vi "observerRegistry.vi"(7 "Action":T1(ring), 8 "error in":errorcluster, 9 "ObservableValue":variant[](array[variant]), 10 "ObservableName":string[](array[string])) -> (0 "error out":errorcluster, 3 "Observable out":T2(c390), 4 "size":i32)   [LabVIEW 2025, in "ObserverClass.lvlib"]
doc: "Handle Observer for each ObservableData available in application"
uses:
  ObserverClass.lvlib
  ObserverClass/Controls/observerControl.ctl
  ObserverClass/ObserverClass.lvclass
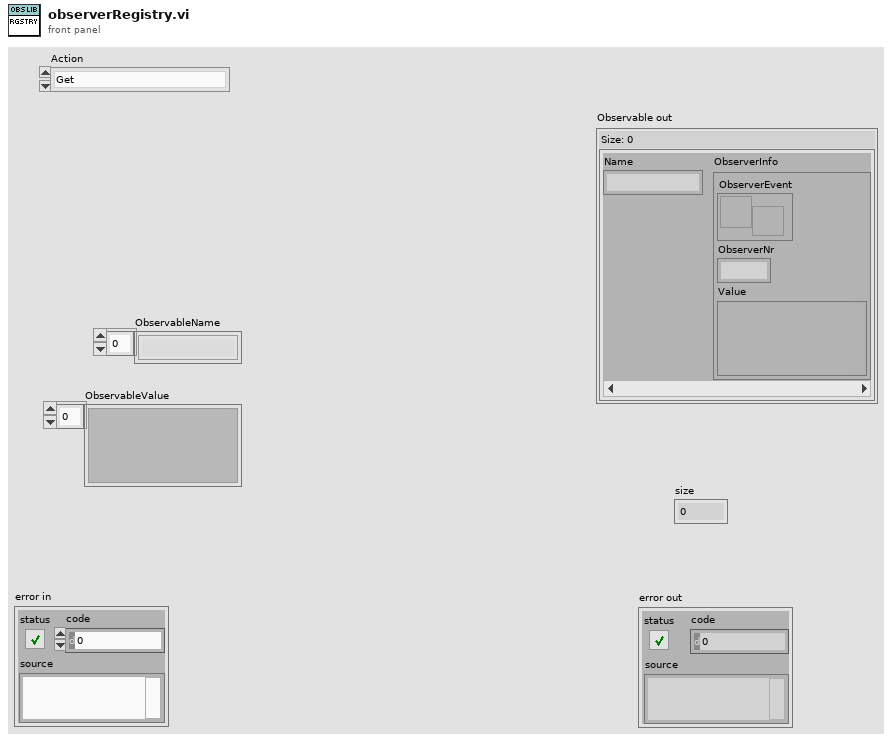
[diagram p1: front panel]
types:
  T1 = enum16{"Get", "Set", "Init", "Remove", "Destroy"}
  T2 = map{string, cluster{"ObserverEvent":refnum<user-event>, "ObserverNr":u64, "Value":variant}}
  T3 = cluster{"ObserverEvent":refnum<user-event>, "ObserverNr":u64, "Value":variant}
  T4 = typedef "ObserverClass.lvlib/ObserverClass.lvclass/observerControl.ctl" = cluster{"ObservableName":string, "ObservableValue":variant, "SenderName":string}
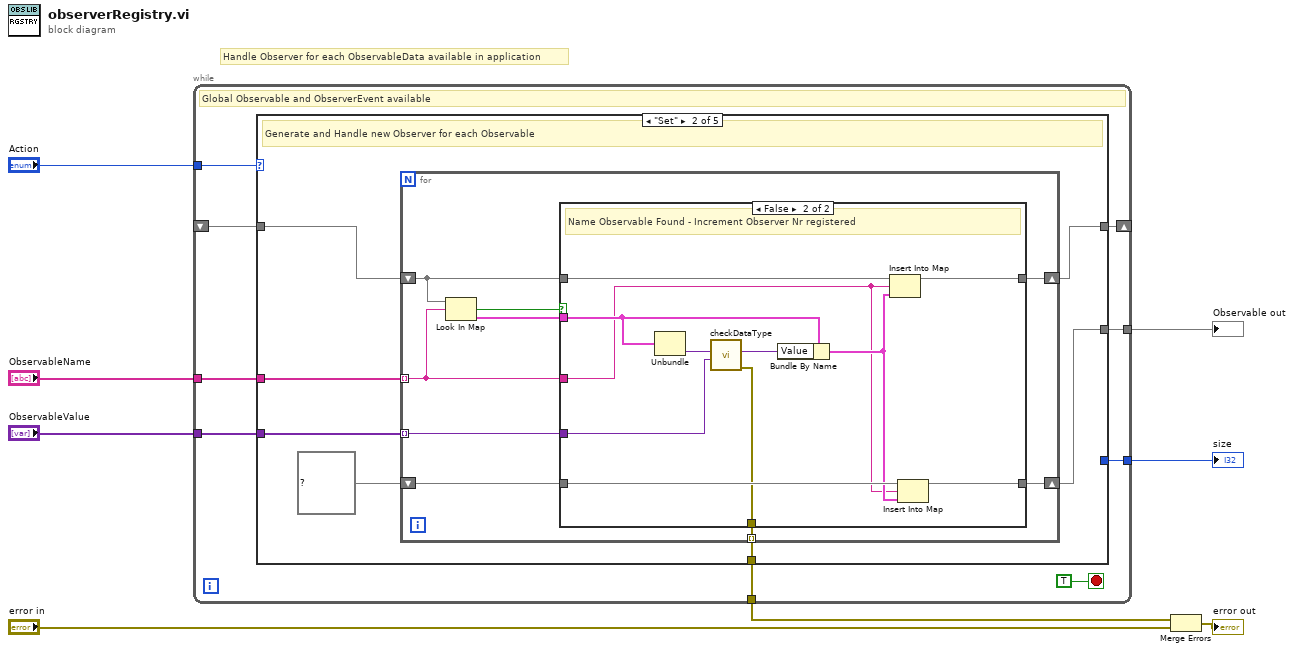
[diagram p0: block diagram]
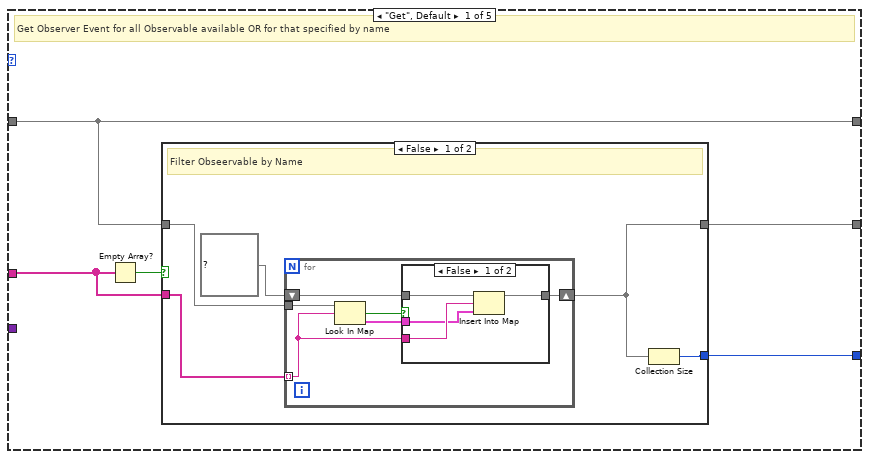
[diagram p2: hidden frame]
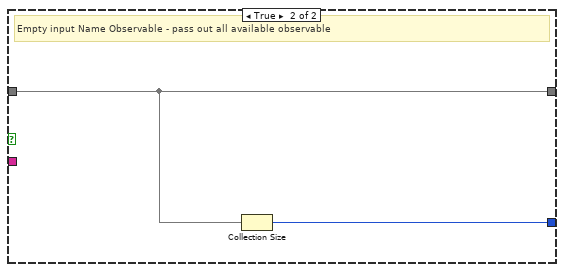
[diagram p4: hidden frame]
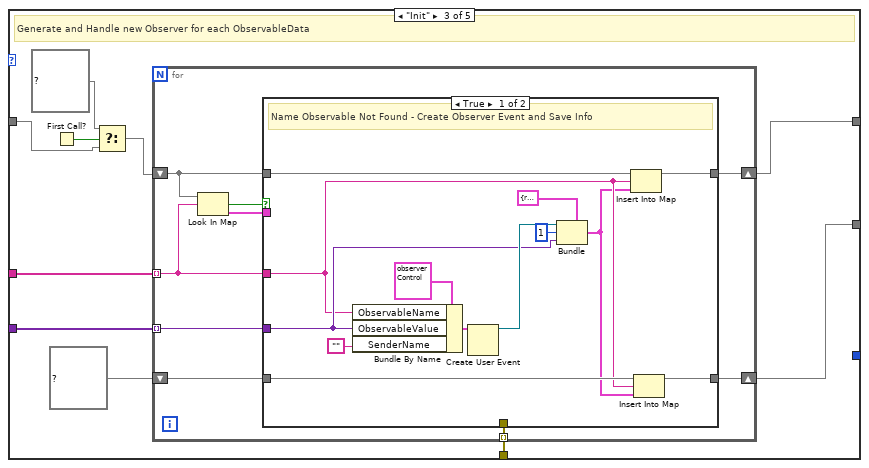
[diagram p6: hidden frame]
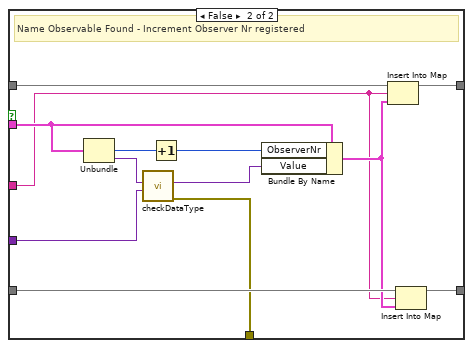
[diagram p7: hidden frame]
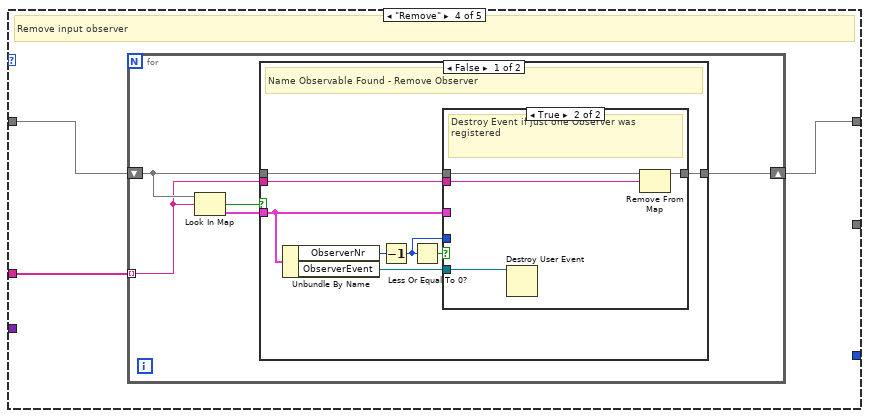
[diagram p8: hidden frame]
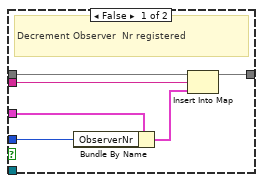
[diagram p9: hidden frame]
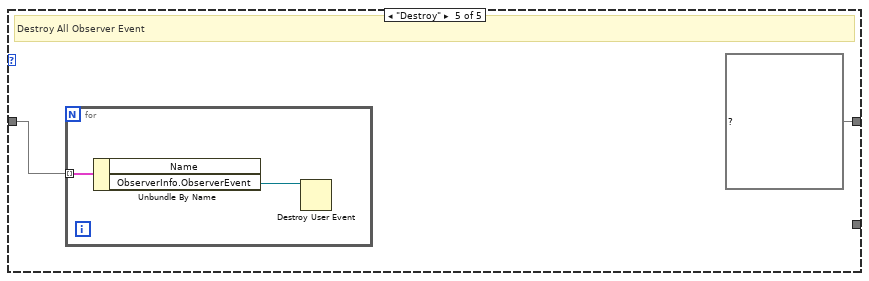
[diagram p11: hidden frame]
diagram:
  # "Handle Observer for each ObservableData available in application"
  n1 = while {
    tunnel: "ObservableName" -> [w17]
    tunnel: "ObservableValue" -> [w16]
    shift-right: [w13] -> _
    shift-left: _ -> [w14]
    tunnel: "Action" -> [w12]
    tunnel: [w11] -> w8
    tunnel: [w10] -> w3
    tunnel: [w9] -> w1
    stop <- TRUE stop-if-true
    # "Global Observable and ObserverEvent available"
    n2 = case shown="\"Set\"" w12 {
      tunnel: w17 -> [w20 w47 w79 w115 _]
      tunnel: w16 -> [_ w46 w78 _ _]
      tunnel: w14 -> [w19 w43 w72 w117 w143]
      tunnel: [w19 w45 w77 w116 T2 {} ("LiveData")] -> w13
      tunnel: [w22 _ _ _ _] -> w11
      tunnel: [w18 w44 w76 _ _] -> w10
      tunnel: [_ w41 w70 _ _] -> w9
      frame "Get", Default {
        # "Get Observer Event for all Observable available OR for that specified by name"
        n3 = Empty Array?(array=w20) -> (empty?=w21:bool)
        n4 = case shown="False" w21 {
          tunnel: [w25 w40] -> w22
          tunnel: w19 -> [w27 w39]
          tunnel: w20 -> [w26 _]
          tunnel: [w24 w39] -> w18
          frame False {
            # "Filter Obseervable by Name"
            n5 = for {
              tunnel: w26 -> [w32] mode=indexing
              tunnel: w27 -> [w33]
              shift-right: [w30] -> w24
              shift-left: T2 {} ("LiveData") -> [w29]
              n6 = Look In Map(map=w33, key=w32) -> (key not found?=w28:bool, value=w31:T3)  [unwired: 1 in]
              n7 = case shown="False" w28 {
                tunnel: w32 -> [w37 _]
                tunnel: w31 -> [w36 _]
                tunnel: [w35 w38] -> w30
                tunnel: w29 -> [w34 w38]
                frame False {
                  n8 = Insert Into Map(map in=w34, key=w37, value=w36) -> (map out=w35:T2)  [unwired: 2 out]
                }
                frame True {
                }
              }
            }
            n9 = Collection Size(1:w24) -> (0:w25:i32)
          }
          frame True {
            # "Empty input Name Observable - pass out all available observable"
            n10 = Collection Size(1:w39) -> (0:w40:i32)
          }
        }
      }
      frame "Set" {
        # "Generate and Handle new Observer for each Observable"
        n11 = for {
          tunnel: w47 -> [w53] mode=indexing
          tunnel: w46 -> [w56] mode=indexing
          shift-right: [w55] -> w45
          shift-left: w43 -> [w54]
          shift-right: [w49] -> w44
          shift-left: T2 {} ("LiveData") -> [w50]
          tunnel: [w48] -> w41 mode=indexing
          n12 = Look In Map(map=w54, key=w53) -> (key not found?=w52:bool, value=w51:T3)  [unwired: 1 in]
          n13 = case shown="False" w52 {
            tunnel: w56 -> [_ w60]
            tunnel: [w58 w67] -> w55
            tunnel: w54 -> [w58 w69]
            tunnel: w53 -> [_ w63]
            tunnel: w51 -> [_ w68]
            tunnel: w50 -> [w57 w66]
            tunnel: [w57 w65] -> w49
            tunnel: [_ w59] -> w48
            frame True {
              # "Name Observable Not Found - Do Nothing"
            }
            frame False {
              # "Name Observable Found - Increment Observer Nr registered"
              n14 = Unbundle(w68) -> ("Value"=w61:variant)  [unwired: 2 out]
              n15 = call "checkDataType.vi"("Data"=w60, "DataType"=w61) -> ("error out"=w59:errorcluster, "Data out"=w62:variant)  [unwired: 8 in]
              n16 = Bundle By Name(cluster=w68, "Value"=w62) -> (w64:T3)
              n17 = Insert Into Map(map in=w69, key=w63, value=w64) -> (map out=w67:T2)  [unwired: 2 out]
              n18 = Insert Into Map(map in=w66, key=w63, value=w64) -> (map out=w65:T2)  [unwired: 2 out]
            }
          }
        }
      }
      frame "Init" {
        # "Generate and Handle new Observer for each ObservableData"
        n19 = First Call?() -> (First Call?: T/F=w75:bool)
        n20 = Select(t=T2 {} ("LiveData"), s=w75, f=w72) -> (s? t:f=w73:T2)
        n21 = for {
          tunnel: w79 -> [w85] mode=indexing
          tunnel: w78 -> [w88] mode=indexing
          shift-right: [w87] -> w77
          shift-left: w73 -> [w86]
          shift-right: [w81] -> w76
          shift-left: T2 {} ("LiveData") -> [w82]
          tunnel: [w80] -> w70 mode=indexing
          n22 = Look In Map(map=w86, key=w85) -> (key not found?=w84:bool, value=w83:T3)  [unwired: 1 in]
          n23 = case shown="True" w84 {
            tunnel: w88 -> [w94 w103]
            tunnel: [w93 w110] -> w87
            tunnel: w86 -> [w98 w114]
            tunnel: w85 -> [w90 w106]
            tunnel: w83 -> [_ w113]
            tunnel: w82 -> [w92 w109]
            tunnel: [w91 w108] -> w81
            tunnel: [_ w102] -> w80
            frame True {
              # "Name Observable Not Found - Create Observer Event and Save Info"
              n24 = Bundle By Name(cluster=T4 {"ObservableName"="", "ObservableValue"=variant, "SenderName"=""} ("Observer"), "ObservableName"=w90, "ObservableValue"=w94, "SenderName"="") -> (w101:T4)
              n25 = Create User Event(user event datatype=w101) -> (user event=w97:refnum<user-event>)  [unwired: 1 in, 1 out]
              n26 = Bundle(cluster=T3 {"ObserverEvent"=refnum, "ObserverNr"=0, "Value"=variant} ("value"), "ObserverEvent"=w97, "ObserverNr"=u64 1, "Value"=w94) -> (w89:T3)
              n27 = Insert Into Map(map in=w98, key=w90, value=w89) -> (map out=w93:T2)  [unwired: 2 out]
              n28 = Insert Into Map(map in=w92, key=w90, value=w89) -> (map out=w91:T2)  [unwired: 2 out]
            }
            frame False {
              # "Name Observable Found - Increment Observer Nr registered"
              n29 = Unbundle(w113) -> ("ObserverNr"=w112:u64, "Value"=w104:variant)  [unwired: 1 out]
              n30 = call "checkDataType.vi"("Data"=w103, "DataType"=w104) -> ("error out"=w102:errorcluster, "Data out"=w105:variant)  [unwired: 8 in]
              n31 = Increment(x=w112) -> (x+1=w111:u64)
              n32 = Bundle By Name(cluster=w113, "ObserverNr"=w111, "Value"=w105) -> (w107:T3)
              n33 = Insert Into Map(map in=w114, key=w106, value=w107) -> (map out=w110:T2)  [unwired: 2 out]
              n34 = Insert Into Map(map in=w109, key=w106, value=w107) -> (map out=w108:T2)  [unwired: 2 out]
            }
          }
        }
      }
      frame "Remove" {
        # "Remove input observer"
        n35 = for {
          shift-right: [w122] -> w116
          shift-left: w117 -> [w121]
          tunnel: w115 -> [w120] mode=indexing
          n36 = Look In Map(map=w121, key=w120) -> (key not found?=w118:bool, value=w119:T3)  [unwired: 1 in]
          n37 = case shown="False" w118 {
            tunnel: [w130 w141] -> w122
            tunnel: w121 -> [w129 w141]
            tunnel: w120 -> [w127 _]
            tunnel: w119 -> [w125 _]
            frame False {
              # "Name Observable Found - Remove Observer"
              n38 = Unbundle By Name(w125) -> ("ObserverNr"=w124:u64, "ObserverEvent"=w128:refnum<user-event>)
              n39 = Decrement(x=w124) -> (x-1=w123:u64)
              n40 = Less Or Equal To 0?(x=w123) -> (x <= 0?=w126:bool)
              n41 = case shown="True" w126 {
                tunnel: [w136 w140] -> w130
                tunnel: w129 -> [w135 w139]
                tunnel: w128 -> [_ w138]
                tunnel: w127 -> [w134 w137]
                tunnel: w125 -> [w133 _]
                tunnel: w123 -> [w132 _]
                frame False {
                  # "Decrement Observer  Nr registered"
                  n42 = Bundle By Name(cluster=w133, "ObserverNr"=w132) -> (w131:T3)
                  n43 = Insert Into Map(map in=w135, key=w134, value=w131) -> (map out=w136:T2)  [unwired: 2 out]
                }
                frame True {
                  # "Destroy Event if just one Observer was registered"
                  n44 = Destroy User Event(user event=w138) -> ()  [unwired: 1 in, 1 out]
                  n45 = Remove From Map(10:w137, 11:w139) -> (3:w140:T2)  [unwired: 2 out]
                }
              }
            }
            frame True {
              # "key LiveData Not Found - Do Nothing"
            }
          }
        }
      }
      frame "Destroy" {
        # "Destroy All Observer Event"
        n46 = for {
          tunnel: w143 -> [w144] mode=indexing
          n47 = Unbundle By Name(w144) -> ("ObserverInfo.ObserverEvent"=w145:refnum<user-event>)  [unwired: 1 out]
          n48 = Destroy User Event(user event=w145) -> ()  [unwired: 1 in, 1 out]
        }
      }
    }
  }
  "size" <- w8
  "Observable out" <- w3
  n49 = Merge Errors(w1, "error in") -> (→"error out":errorcluster)
